vi "配置保存写入.vi"(8 "error in (no error)":errorcluster caption="错误输入（无错误）", 11 "配置":enum16{"读取", "写入"}(ring)) -> (0 "error out":errorcluster caption="错误输出")   [LabVIEW 2016, in "main.lvlib"]
uses:
  main.lvlib
  <vilib>/Utility/config.llb/NI_LVConfig.lvlib
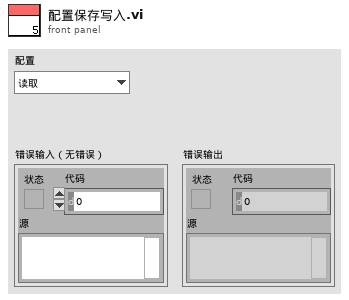
[diagram p1: front panel]
types:
  T1 = typedef "NI_LVConfig.lvlib/Config Data RefNum.ctl" = refnum<k1>
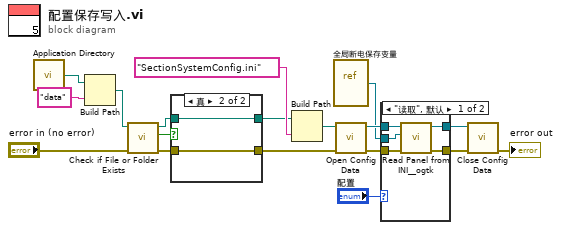
[diagram p0: block diagram]
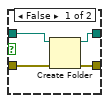
[diagram p2: hidden frame]
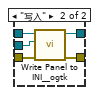
[diagram p3: hidden frame]
diagram:
  n1 = call <vilib>:"Application Directory.vi"() -> ("Application Directory"=w14:path)
  n2 = Build Path(base path=w14, name or relative path="data" ("名称或相对路径")) -> (appended path=w7:path)
  n3 = call <vilib>:"Check if File or Folder Exists.vi"("error in (no error)"="error in (no error)", "path"=w7) -> ("error out"=w3:errorcluster, "file or folder exists?"=w5:bool, "dup path"=w4:path)  [unwired: 7 in]
  n4 = case shown="真" w5 {
    tunnel: [w21 w24] -> w1
    tunnel: w4 -> [w22 w24]
    tunnel: w3 -> [w20 w23]
    tunnel: [w19 w23] -> w2
    frame False {
      n5 = Create Folder(path (use dialog)=w22, error in=w20) -> (created path=w21:path, error out=w19:errorcluster)  [unwired: 1 in, 1 out]
    }
    frame True {
    }
  }
  n6 = Build Path(base path=w1, name or relative path="SectionSystemConfig.ini" ("名称或相对路径")) -> (appended path=w12:path)
  n7 = vi-ref "全局断电保存变量.vi"() -> (w10:refnum<vi>)
  n8 = call <vilib>:"Open Config Data.vi"("error in (no error)"=w2, "configuration file path"=w12) -> ("error out"=w15:errorcluster, "refnum"=w18:T1)  [unwired: 7 in, 1 out]
  n9 = case shown="\"读取\", 默认" "配置" {
    tunnel: w18 -> [w27 w34]
    tunnel: [w25 w33] -> w17
    tunnel: [w28 w32] -> w16
    tunnel: w15 -> [w29 w31]
    tunnel: w10 -> [w26 w30]
    frame "读取", Default {
      n10 = call <userlib>:"Read Panel from INI__ogtk.vi"("error in (no error)"=w29, "VI ref"=w26, "refnum"=w27) -> ("error out"=w28:errorcluster, "refnum out"=w25:T1)  [unwired: 7 in]
    }
    frame "写入" {
      n11 = call <userlib>:"Write Panel to INI__ogtk.vi"("error in (no error)"=w31, "VI ref"=w30, "refnum"=w34) -> ("error out"=w32:errorcluster, "refnum out"=w33:T1)  [unwired: 7 in]
    }
  }
  n12 = call <vilib>:"Close Config Data.vi"("error in (no error)"=w16, "refnum"=w17) -> ("error out"=→"error out":errorcluster)  [unwired: 8 in, 1 out]
